vi "PSO_UpdateVelocities.vi"(8 "Parameters in":T2={"Swarm size"=0, "Generations no."=0, "Cognitive coeff a1"=0.0, "Social coeff a2"=0.0, "Min inertia weight"=0.0, "Max inertia weight "=0.9, "Fmax"=0} {"Generations no." min=1; "Swarm size" min=1}, 9 "Generation":i32, 10 "Gbest Particle":i32[](array[numeric]), 11 "Population":T1) -> (2 "Inertia Weight":dbl, 3 "Population out":T1)   [LabVIEW 2016, in "Optimal Frequency Bands Search.lvlib" / "ParticleSwarm.lvlib"]
doc: "Рассчитать новые векторы скорости для всех частиц роя."
uses:
  ParticleSwarm.lvlib
  PSO_tPopulation.ctl
  PSO_tParameters.ctl
panel:
  # "This VI is a part of BCI Design library, http://www.ru-bci.org \nCopyright © 2020, Sotnikov Peter, All rights reserved. License: GNU GPLv3"
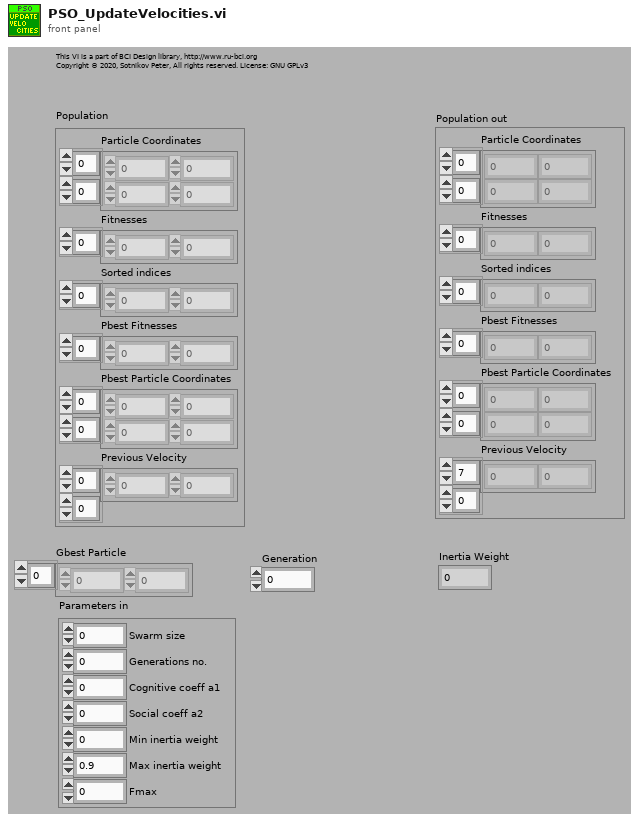
[diagram p1: front panel]
types:
  T1 = typedef "Optimal Frequency Bands Search.lvlib/ParticleSwarm.lvlib/PSO_tPopulation.ctl" = cluster{"Particle Coordinates":i32[][], "Fitnesses":dbl[], "Sorted indices":i32[], "Pbest Fitnesses":dbl[], "Pbest Particle Coordinates":i32[][], "Previous Velocity":dbl[][]}
  T2 = typedef "Optimal Frequency Bands Search.lvlib/ParticleSwarm.lvlib/PSO_tParameters.ctl" = cluster{"Swarm size":i32, "Generations no.":i32, "Cognitive coeff a1":dbl, "Social coeff a2":dbl, "Min inertia weight":dbl, "Max inertia weight ":dbl, "Fmax":i32}
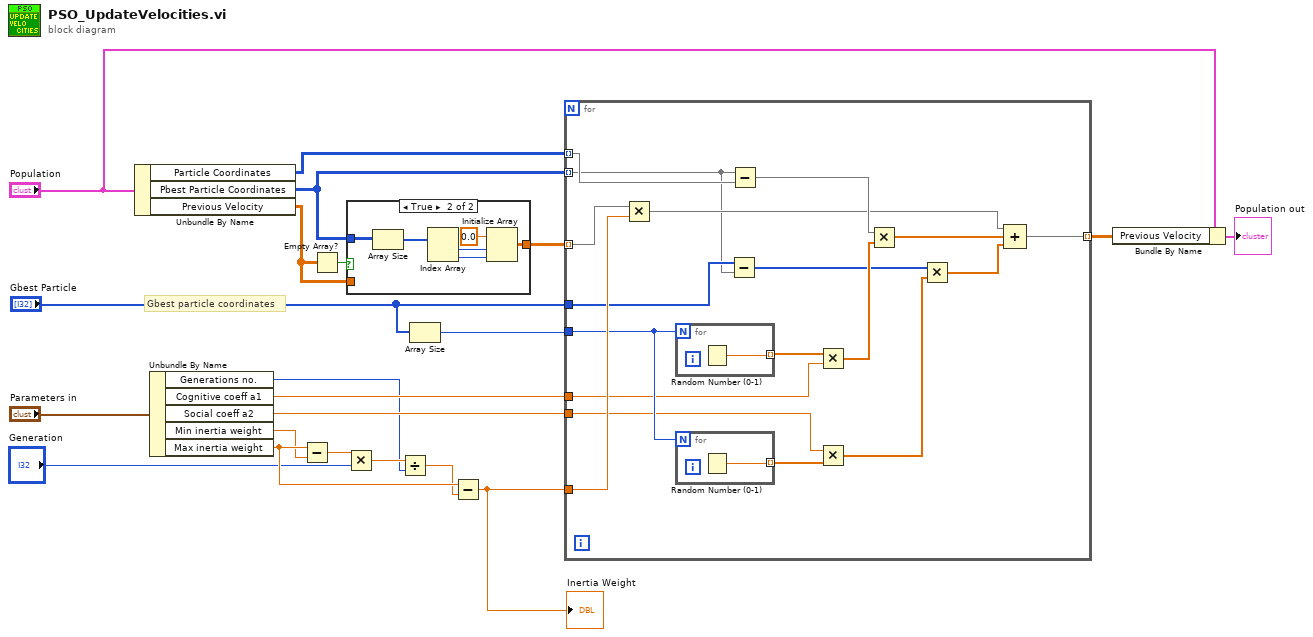
[diagram p0: block diagram]
diagram:
  # "Gbest particle coordinates"
  n1 = Unbundle By Name("Population") -> ("Particle Coordinates"=w21:i32[][], "Pbest Particle Coordinates"=w4:i32[][], "Previous Velocity"=w2:dbl[][])
  n2 = Unbundle By Name("Parameters in") -> ("Generations no."=w12:i32, "Cognitive coeff a1"=w19:dbl, "Social coeff a2"=w18:dbl, "Min inertia weight"=w16:dbl, "Max inertia weight"=w17:dbl)
  n3 = Subtract(x=w17, y=w16) -> (x-y=w15:dbl)
  n4 = Empty Array?(array=w2) -> (empty?=w3:bool)
  n5 = Multiply(x=w15, y="Generation") -> (x*y=w13:dbl)
  n6 = case shown="True" w3 {
    tunnel: w4 -> [_ w28]
    tunnel: w2 -> [w22 _]
    tunnel: [w22 w23] -> w1
    frame False {
    }
    frame True {
      n7 = Array Size(array=w28) -> (size(s)=w27:i32[])
      n8 = Index Array(array=w27) -> (element #1=w25:i32, element #2=w26:i32)  [unwired: 2 in]
      n9 = Initialize Array(0.0 ("element"), w25, w26) -> (w23:dbl[][])
    }
  }
  n10 = Divide(x=w13, y=w12) -> (x/y=w11:dbl)
  n11 = Array Size(array="Gbest Particle") -> (size(s)=w8:i32)
  n12 = Subtract(x=w17, y=w11) -> (x-y=w10:dbl)
  "Inertia Weight" <- w10
  n13 = for {
    tunnel: w21 -> [w31] mode=indexing
    tunnel: w4 -> [w29] mode=indexing
    tunnel: "Gbest Particle" -> [w30]
    tunnel: w19 -> [w43]
    tunnel: w18 -> [w41]
    tunnel: w10 -> [w46]
    tunnel: w8 -> [w45]
    tunnel: [w33] -> w6 mode=indexing
    tunnel: w1 -> [w32] mode=indexing
    n14 = Multiply(x=w32, y=w46) -> (x*y=w36:dbl[])
    n15 = for {
      N: w45 -> [_]
      tunnel: [w48] -> w44 mode=indexing
      n16 = Random Number (0-1)() -> (number: 0 to 1=w48:dbl)
    }
    n17 = for {
      N: w45 -> [_]
      tunnel: [w47] -> w42 mode=indexing
      n18 = Random Number (0-1)() -> (number: 0 to 1=w47:dbl)
    }
    n19 = Subtract(x=w30, y=w29) -> (x-y=w38:i32[])
    n20 = Subtract(x=w29, y=w31) -> (x-y=w40:i32[])
    n21 = Multiply(x=w44, y=w43) -> (x*y=w39:dbl[])
    n22 = Multiply(x=w41, y=w42) -> (x*y=w37:dbl[])
    n23 = Multiply(x=w40, y=w39) -> (x*y=w35:dbl[])
    n24 = Multiply(x=w38, y=w37) -> (x*y=w34:dbl[])
    n25 = Compound Arithmetic op=ADD(w36, w35, w34) -> (w33:dbl[])
  }
  n26 = Bundle By Name(cluster="Population", "Previous Velocity"=w6) -> (→"Population out":T1)
